vi "Auto-Refresh Read.vi"(8 "error in (no error)":errorcluster, 11 "SimSyA in":refnum<class "SimSyA.lvclass">) -> (0 "error out":errorcluster, 1 "Control Data":T1, 2 "1 Sample":T2, 3 "SimSyA out":refnum<class "SimSyA.lvclass">)   [LabVIEW 2014, in "SimSyA.lvlib" / "SimSyA.lvclass"]
uses:
  SimSyA.lvclass
  DriverMasterSync/build/DriverMasterSync.lvlibp/APIs/Data Queue/Acquisition Data 1 Sample Cluster.ctl
  DriverMasterSync/build/DriverMasterSync.lvlibp/APIs/Data Queue/Control Data Cluster.ctl
  SimSyA.lvclass/SimSyA.ctl
  DriverMasterSync/build/DriverMasterSync.lvlibp/Modules/HAL/DriverMasterSync/DriverMasterSyncClass/DriverMasterSync.lvclass
  SimSyA.lvlib
  DriverMasterSync/build/DriverMasterSync.lvlibp/APIs/Data Queue/WINFAS 2 Data Queue.lvlib
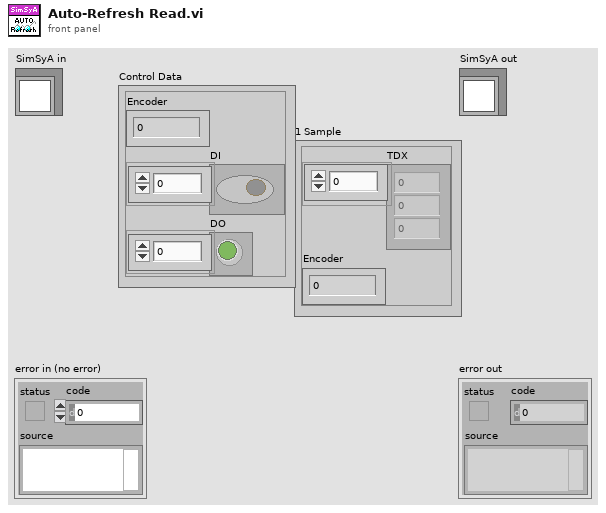
[diagram p1: front panel]
types:
  T1 = typedef "DriverMasterSync.lvlibp/WINFAS 2 Data Queue.lvlib/Control Data Cluster.ctl" = cluster{"Encoder":sgl, "DI":bool[], "DO":bool[]}
  T2 = typedef "DriverMasterSync.lvlibp/WINFAS 2 Data Queue.lvlib/Acquisition Data 1 Sample Cluster.ctl" = cluster{"TDX":sgl[], "Encoder":sgl}
  T3 = cluster{"TDX":sgl[], "Encoder":i32, "DI Counter":u32, "DO Mask":u32}
  T4 = typedef "DriverMasterSync.lvlibp/WINFAS 2 Data Queue.lvlib/Acquisition Data Cluster.ctl" = T2[]
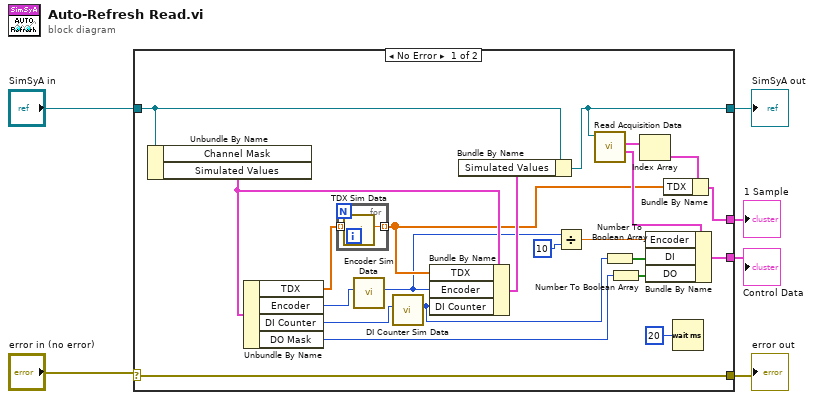
[diagram p0: block diagram]
diagram:
  n1 = case shown="No Error" "error in (no error)" {
    selector: "error in (no error)" -> [w28 w32]
    tunnel: [w28 w32] -> w5
    tunnel: [w19 w31] -> w3
    tunnel: "SimSyA in" -> [w20 w31]
    tunnel: [w25 _] -> w2
    tunnel: [w23 _] -> w1
    frame No Error {
      n2 = Unbundle By Name(w20) -> ("Simulated Values"=w18:T3)  [unwired: 1 out]
      n3 = Unbundle By Name(w18) -> ("TDX"=w13:sgl[], "Encoder"=w14:i32, "DI Counter"=w15:u32, "DO Mask"=w21:u32)
      n4 = for {
        tunnel: w13 -> [w30] mode=indexing
        tunnel: [w29] -> w12 mode=indexing
        n5 = call "TDX Sim Data.vi"("TDX in"=w30) -> ("TDX out"=w29:sgl)  [unwired: 10 in]
      }
      n6 = call "Encoder Sim Data.vi"("Encoder in"=w14) -> ("Encoder out"=w9:i32)  [unwired: 10 in]
      n7 = call "DI Counter Sim Data.vi"("DI Counter in"=w15) -> ("DI Counter out"=w10:u32)  [unwired: 10 in]
      n8 = Bundle By Name(cluster=w18, "TDX"=w12, "Encoder"=w9, "DI Counter"=w10) -> (w17:T3)
      n9 = Bundle By Name(cluster=w20, "Simulated Values"=w17) -> (w19:refnum<class "SimSyA.lvclass">)
      n10 = Divide(x=w9, y=10) -> (x/y=w7:dbl)
      n11 = call "Read Acquisition Data.vi"("DriverMasterSync in"=w19) -> ("Control Data"=w24:T1, "Acquisition Data"=w27:T4)  [unwired: 7 in, 2 out]
      n12 = Number To Boolean Array(number=w10) -> (Boolean array=w11:bool[])
      n13 = Number To Boolean Array(number=w21) -> (Boolean array=w22:bool[])
      n14 = Index Array(array=w27) -> (element=w26:T2)  [unwired: 1 in]
      n15 = Bundle By Name(cluster=w24, "Encoder"=w7, "DI"=w11, "DO"=w22) -> (w23:T1)
      n16 = Bundle By Name(cluster=w26, "TDX"=w12) -> (w25:T2)
      n17 = Wait (ms)(milliseconds to wait=u32 20) -> ()  [unwired: 1 out]
    }
    frame Error {
    }
  }
  "error out" <- w5
  "SimSyA out" <- w3
  "1 Sample" <- w2
  "Control Data" <- w1
